vi "terminate.vi"(8 "error in (no error)":errorcluster, 11 "DL090215DataCollection in":refnum<class "DataCollectionDL090215.lvclass">) -> (0 "error out":errorcluster, 3 "DL090215DataCollection out":refnum<class "DataCollectionDL090215.lvclass">)   [LabVIEW 2010, in "DataCollectionDL090215.lvclass"]
uses:
  DataCollectionDL090215.lvclass
  DataCollectionDL091104Scaffold/DataCollectionDL091104Scaffold/DataCollectionDL091104Scaffold.lvclass
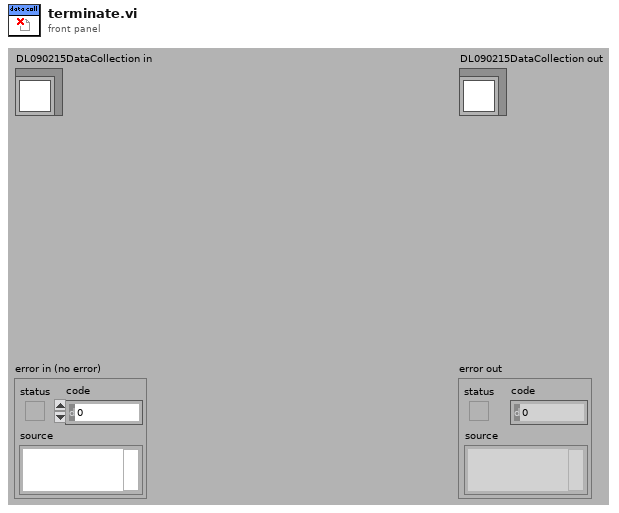
[diagram p1: front panel]
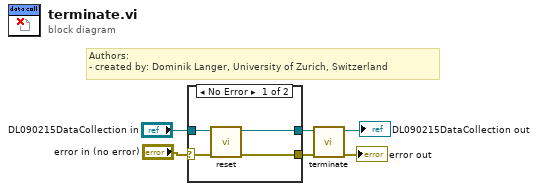
[diagram p0: block diagram]
diagram:
  # "Authors: \n- created by: Dominik Langer, University of Zurich, Switzerland"
  n1 = case shown="No Error" "error in (no error)" {
    selector: "error in (no error)" -> [w8 w12]
    tunnel: [w7 w12] -> w4
    tunnel: [w9 w11] -> w3
    tunnel: "DL090215DataCollection in" -> [w10 w11]
    frame No Error {
      n2 = call-dynamic "reset.vi"("error in (no error)"=w8, "DL090215DataCollection in"=w10) -> ("error out"=w7:errorcluster, "DL090215DataCollection out"=w9:refnum<class "DataCollectionDL090215.lvclass">)  [unwired: 8 in]
    }
    frame Error {
    }
  }
  n3 = call-parent "terminate.vi"("error in (no error)"=w4, "GenericPlugin in"=w3) -> ("error out"=→"error out":errorcluster, "GenericPlugin out"=→"DL090215DataCollection out":refnum<class "DataCollectionDL090215.lvclass">)  [unwired: 8 in]
